vi "Autolocate Fiducials.vi"(6 "FD Index":i32, 8 "error in":errorcluster, 9 "Past Fiducials":dbl[](array[numeric]), 10 "Component":T1, 11 "Gantry In":refnum<k24>) -> (0 "error out":errorcluster, 1 "Wrong Orientation?":bool, 2 "Component Out":T1, 3 "Gantry Out":refnum<k24>)   [LabVIEW 2021, in "Component Tray.lvclass"]
uses:
  Component Tray.lvclass
  C:/Program Files (x86)/Aerotech/A3200/LabVIEW/2010/Bin/Aerotech.A3200.dll
  Program Files (x86)/Aerotech/A3200/LabVIEW/2010/Bin/Aerotech.A3200.dll
  Find Component.ctl
  Controller/Camera/Machine Vision.ctl
  Controller/Motion/A3200/A3200.lvclass
  Controller/Motion/Motion.lvclass
  Controller/Camera/Camera.lvclass
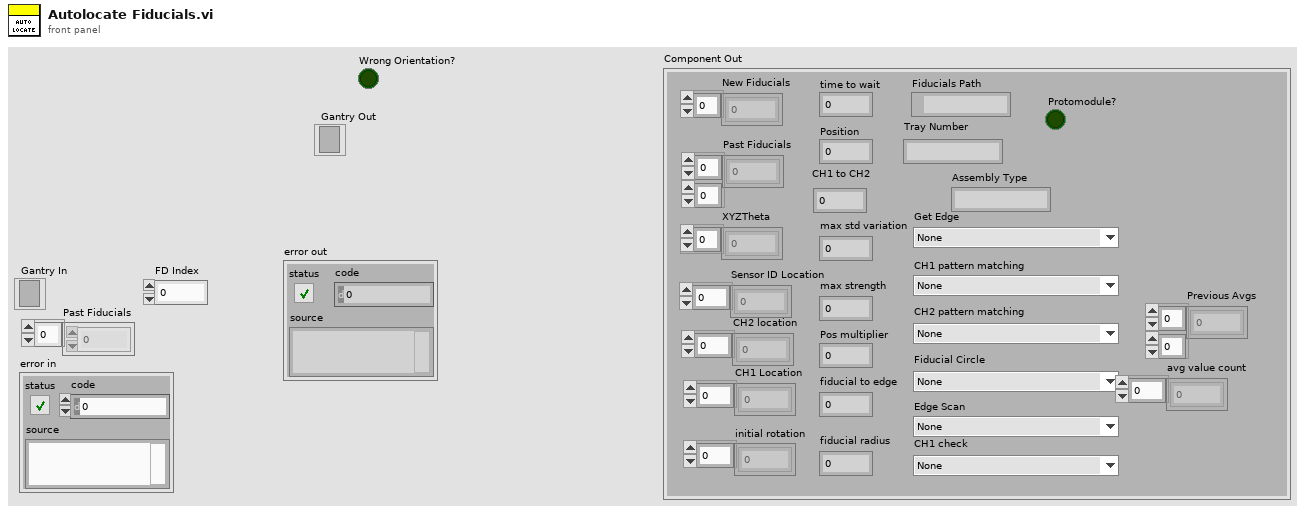
[diagram p1: front panel]
types:
  T1 = typedef "Component Tray.lvclass/Find Component.ctl" = cluster{"New Fiducials":dbl[], "Past Fiducials":dbl[][], "XYZTheta":dbl[], "Fiducials Path":path, "Position":i32, "CH1 Location":dbl[], "Sensor ID Location":dbl[], "initial rotation":dbl[], "CH2 location":dbl[], "max std variation":dbl, "max strength":dbl, "CH2 pattern matching":T2, "Fiducial Circle":T2, "Get Edge":T2, "Pos multiplier":dbl, "time to wait":u32, "fiducial to edge":dbl, "Protomodule?":bool, "Assembly Type":string, "CH1 to CH2":dbl, "Tray Number":string, "fiducial radius":dbl, "4 fiducials?":bool, "CH1 check":T2, "Edge Scan":T2, "CH1 pattern matching":T2, "Sensor Thickness":dbl, "Previous Avgs":dbl[][], "avg value count":dbl[]}
  T2 = typedef "Camera.lvclass/Machine Vision.ctl" = enum16{"None", "Assembly Tray Circle", "Assembly Tray Fiducial", "Partial Hexaboard", "sensor edge init", "HB edge init", "sensor edge pos1", "sensor edge pos2", "HB edge pos1", "HB edge pos2", "Sensor CH1-2", "HB CH1", "HB CH2", "V3 Sensor Circle", "Hexaboard Circle", "sensor CH1 check", "HB CH1 check ", "sensor ID"}
  T3 = enum16{"None", "Assembly Tray Circle", "Assembly Tray Fiducial", "Partial Hexaboard", "sensor edge init", "HB edge init", "sensor edge pos1", "sensor edge pos2", "HB edge pos1", "HB edge pos2", "Sensor CH1-2", "HB CH1", "HB CH2", "V3 Sensor Circle", "Hexaboard Circle", "sensor CH1 check", "HB CH1 check "}
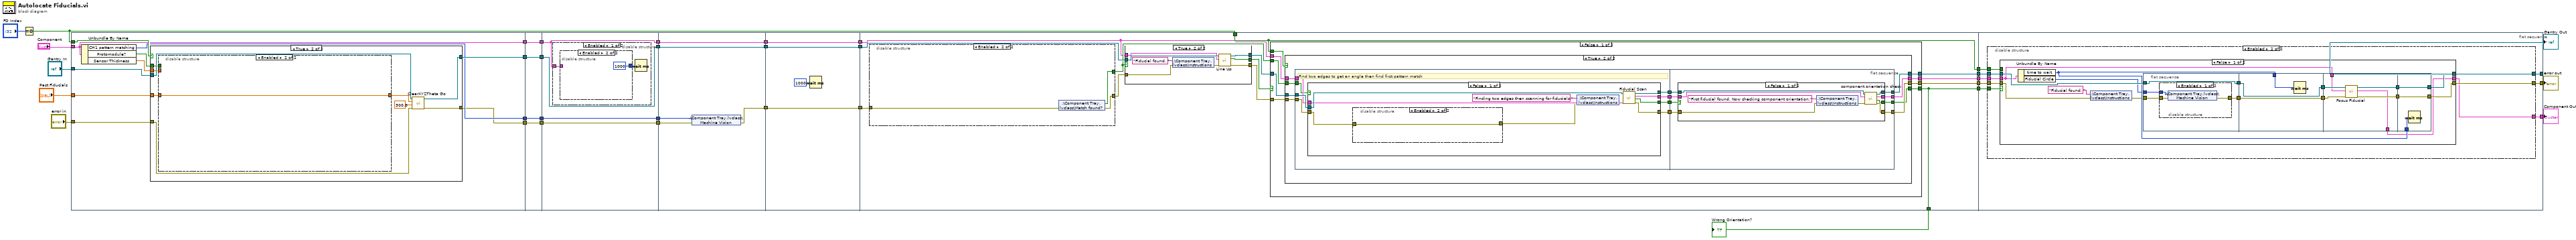
[diagram p0: block diagram]
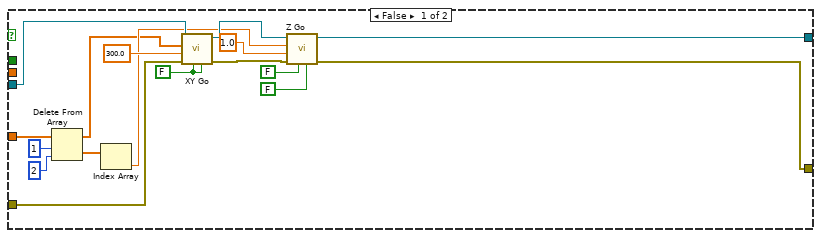
[diagram p2: hidden frame]
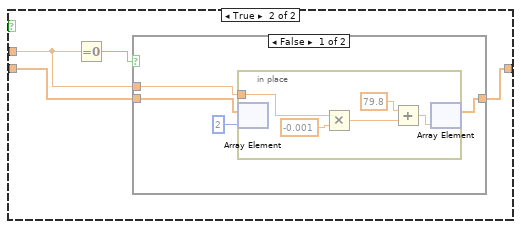
[diagram p4: hidden frame]
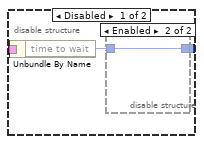
[diagram p6: hidden frame]
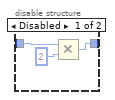
[diagram p7: hidden frame]
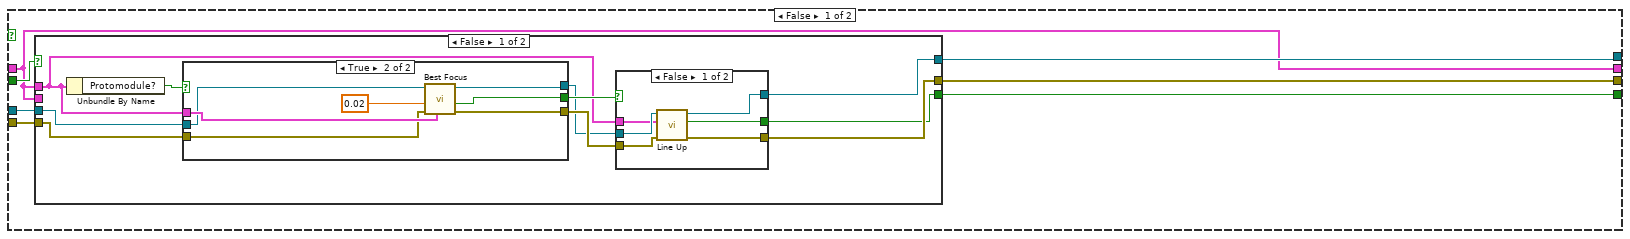
[diagram p9: hidden frame]
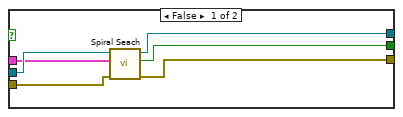
[diagram p10: hidden frame]
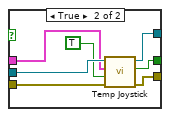
[diagram p11: hidden frame]
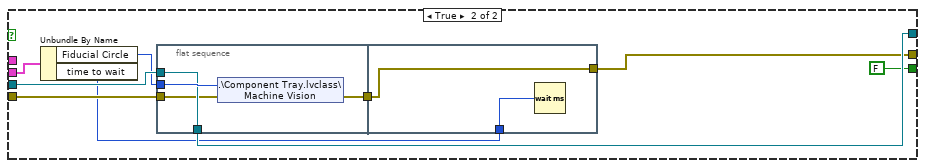
[diagram p12: hidden frame]
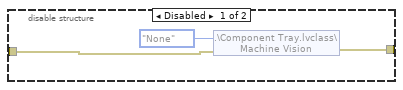
[diagram p13: hidden frame]
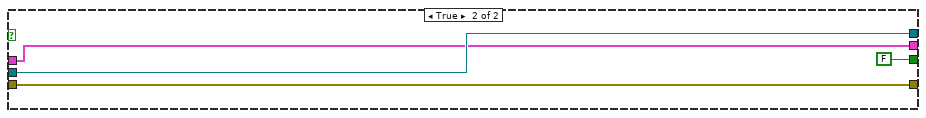
[diagram p14: hidden frame]
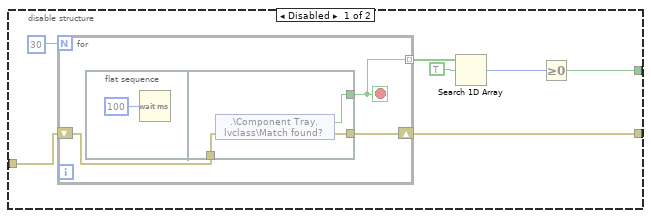
[diagram p17: hidden frame]
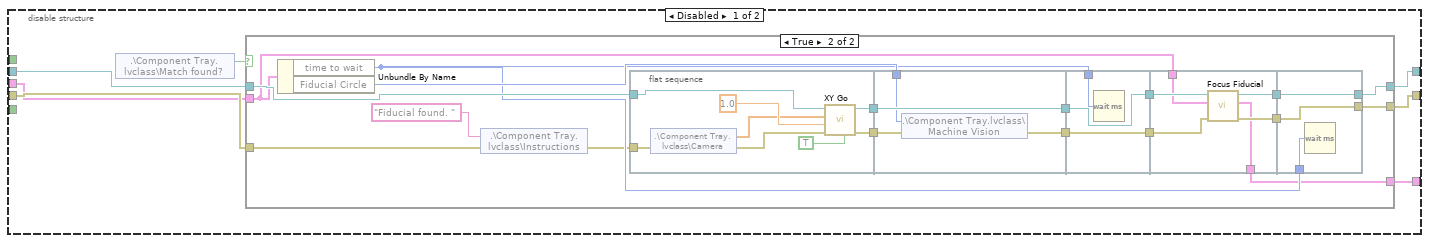
[diagram p19: hidden frame]
diagram:
  n1 = Equal To 0?(x="FD Index") -> (x = 0?=w29:bool)
  n2 = flat-sequence {
    tunnel: w29 -> [w43]
    tunnel: "Gantry In" -> [w42]
    tunnel: "Past Fiducials" -> [w41]
    tunnel: "error in" -> [w36]
    tunnel: [w40] -> w16
    tunnel: "Component" -> [w39]
    tunnel: [w39] -> w18
    tunnel: [w35] -> w10
    tunnel: [w34] -> w7
    tunnel: w18 -> [w93]
    tunnel: [w93] -> w17
    tunnel: w16 -> [w92]
    tunnel: [w92] -> w15
    tunnel: [w91] -> w11
    tunnel: w10 -> [w91]
    tunnel: [w90] -> w8
    tunnel: w7 -> [w90]
    tunnel: w17 -> [w97]
    tunnel: [w97] -> w13
    tunnel: w15 -> [w96]
    tunnel: [w96] -> w14
    tunnel: [w95] -> w12
    tunnel: w11 -> [w95]
    tunnel: [w94] -> w9
    tunnel: w8 -> [w94]
    tunnel: w14 -> [w112]
    tunnel: [w112] -> w6
    tunnel: [w108] -> w4
    tunnel: w13 -> [w111]
    tunnel: [w111] -> w2
    tunnel: w12 -> [w110]
    tunnel: w9 -> [w109]
    tunnel: w6 -> [w116]
    tunnel: [w116] -> w5
    tunnel: w4 -> [w115]
    tunnel: [w115] -> w3
    tunnel: w2 -> [w114]
    tunnel: [w114] -> w1
    tunnel: w29 -> [w125]
    tunnel: [w129] -> w28
    tunnel: [w127] -> w27
    tunnel: [w128] -> w25
    tunnel: [w126] -> w24
    tunnel: [w126] -> w23
    tunnel: [w125] -> w22
    tunnel: w5 -> [w121]
    tunnel: w3 -> [w124]
    tunnel: w1 -> [w118]
    tunnel: [w295] -> w19
    tunnel: [w294] -> w21
    tunnel: w28 -> [w293]
    tunnel: w27 -> [w291]
    tunnel: [w290] -> w20
    tunnel: w25 -> [w292]
    tunnel: w23 -> [w289]
    tunnel: w22 -> [w288]
    frame #0 {
      n3 = Unbundle By Name(w39) -> ("CH1 pattern matching"=w35:T2, "Protomodule?"=w38:bool, "Sensor Thickness"=w37:dbl)
      n4 = case shown="True" w43 {
        tunnel: w41 -> [w56 w65]
        tunnel: w42 -> [w60 w69]
        tunnel: [w54 w68] -> w40
        tunnel: w36 -> [w58 w67]
        tunnel: w38 -> [_ w61]
        tunnel: [w53 w66] -> w34
        tunnel: w37 -> [_ w64]
        frame False {
          w59 = FALSE ("Increment?")
          n5 = Delete From Array(array=w56, length=1, index=2) -> (deleted portion=w46:dbl[], array with subset deleted=w44:dbl[])
          n6 = Index Array(array=w46) -> (element=w45:dbl)  [unwired: 1 in]
          n7 = call "XY Go.vi"("Increment?"=w59, "return immediately"=w59, "error in (no error)"=w58, "Speed"=300.0, "XY In"=w44, "Gantry In"=w60) -> ("error out"=w52:errorcluster, "Gantry Out"=w55:refnum<k24>)  [unwired: 3 in, 1 out]
          n8 = call "Z Go.vi"("Increment"=FALSE, "Return Immediately"=FALSE, "error in (no error)"=w52, "Speed In"=1.0, "Position In"=w45, "Gantry In"=w55) -> ("error out"=w53:errorcluster, "Gantry Out"=w54:refnum<k24>)  [unwired: 2 in, 2 out]
        }
        frame True {
          n9 = disable-structure shown="Enabled" {
            disable-tunnel: w65 -> [w73 w89]
            disable-tunnel: w64 -> [w72 _]
            disable-tunnel: [w71 w89] -> w63
            disable-tunnel: w61 -> [w70 _]
            frame Disabled {
              n10 = case shown="False" w70 {
                tunnel: w73 -> [w74 w77]
                tunnel: w72 -> [_ w76]
                tunnel: [w74 w75] -> w71
                frame False {
                }
                frame True {
                  n11 = Equal To 0?(x=w76) -> (x = 0?=w78:bool)
                  n12 = case shown="False" w78 {
                    tunnel: w77 -> [w82 w88]
                    tunnel: w76 -> [w81 _]
                    tunnel: [w80 w88] -> w75
                    frame False {
                      n13 = in-place {
                        in-place-border: w81 -> [w86]
                        n14 = in-place-array #1(w82, 2) -> ()  [unwired: 1 out]
                        n15 = Multiply(x=w86, y=-0.001) -> (x*y=w84:dbl)
                        n16 = Add(x=79.8, y=w84) -> (x+y=w83:dbl)
                        n17 = in-place-array #1(w83) -> (w80:dbl[])  [unwired: 1 out]
                      }
                    }
                    frame True {
                    }
                  }
                }
              }
            }
            frame Enabled {
            }
          }
          n18 = call "ClearXYZTheta Go.vi"("error in (no error)"=w67, "Speed"=300.0, "XYZTheta In"=w63, "Gantry In"=w69) -> ("error out"=w66:errorcluster, "Gantry Out"=w68:refnum<k24>)  [unwired: 5 in, 1 out]
        }
      }
    }
    frame #1 {
    }
    frame #2 {
      n19 = disable-structure shown="Enabled" {
        disable-tunnel: w97 -> [w99 _]
        frame Enabled {
          n20 = disable-structure shown="Enabled" {
            disable-tunnel: w99 -> [w102 _]
            disable-tunnel: [w100 u32 1000 ("time to wait")] -> w98
            frame Disabled {
              n21 = Unbundle By Name(w102) -> ("time to wait"=w101:u32)
              n22 = disable-structure shown="Enabled" {
                disable-tunnel: w101 -> [w105 w106]
                disable-tunnel: [w103 w106] -> w100
                frame Disabled {
                  n23 = Multiply(x=w105, y=u32 2) -> (x*y=w103:u32)
                }
                frame Enabled {
                }
              }
            }
            frame Enabled {
            }
          }
          n24 = Wait (ms)(milliseconds to wait=w98) -> ()  [unwired: 1 out]
        }
        frame Disabled {
        }
      }
    }
    frame #3 {
      n25 = shared-variable ".\\Component Tray.lvclass\\Machine Vision"(w110, error in=w109) -> (error out=w108:errorcluster)
    }
    frame #4 {
      n26 = Wait (ms)(milliseconds to wait=u32 1000) -> ()  [unwired: 1 out]
    }
    frame #5 {
      n27 = disable-structure shown="Enabled" {
        disable-tunnel: w124 -> [w266 w275]
        disable-tunnel: [w264 w276] -> w123
        disable-tunnel: [w260 w274] -> w119
        frame Disabled {
          n28 = for {
            N: 30 -> [_]
            tunnel: [w268] -> w263 mode=indexing
            shift-right: [w267] -> w264
            shift-left: w266 -> [w269]
            stop <- w268 stop-if-true
            n29 = flat-sequence {
              tunnel: w269 -> [w273]
              tunnel: [w272] -> w268
              tunnel: [w271] -> w267
              frame #0 {
                n30 = Wait (ms)(milliseconds to wait=u32 100) -> ()  [unwired: 1 out]
              }
              frame #1 {
                n31 = shared-variable ".\\Component Tray.lvclass\\Match found?"(error in=w273) -> (w272:bool, error out=w271:errorcluster)
              }
            }
          }
          n32 = Search 1D Array(1D array=w263, element=TRUE) -> (index of element=w261:i32)  [unwired: 1 in]
          n33 = Greater Or Equal To 0?(x=w261) -> (x >= 0?=w260:bool)
        }
        frame Enabled {
          n34 = shared-variable ".\\Component Tray.lvclass\\Match found?"(error in=w275) -> (w274:bool, error out=w276:errorcluster)
        }
      }
      n35 = case shown="True" w119 {
        selector: w119 -> [w277 _]
        tunnel: w123 -> [w279 w286]
        tunnel: [w279 w282] -> w122
        tunnel: w121 -> [w278 w285]
        tunnel: [w278 w284] -> w120
        tunnel: w118 -> [_ w281]
        tunnel: [w277 w280] -> w117
        frame False {
        }
        frame True {
          n36 = shared-variable ".\\Component Tray.lvclass\\Instructions"("Fiducial found. " ("Instructions"), error in=w286) -> (error out=w283:errorcluster)
          n37 = call "Line Up.vi"("error IO"=w283, "Component"=w281, "Gantry In"=w285) -> ("error out"=w282:errorcluster, "Error?"=w280:bool, "Gantry Out"=w284:refnum<k24>)  [unwired: 6 in]
        }
      }
      n38 = case shown="False" w117 {
        selector: w117 -> [_ w257]
        tunnel: [w138 w259] -> w129
        tunnel: [w137 w258] -> w128
        tunnel: [w136 w256] -> w127
        tunnel: [w135 w257] -> w126
        tunnel: w125 -> [w134 _]
        tunnel: w122 -> [w133 w258]
        tunnel: w120 -> [w132 w259]
        tunnel: w119 -> [w131 _]
        tunnel: w118 -> [w130 w256]
        frame False {
          n39 = case shown="True" w134 {
            tunnel: w132 -> [w145 w208]
            tunnel: [w144 w207] -> w138
            tunnel: [w143 w206] -> w137
            tunnel: w130 -> [w139 w205]
            tunnel: [w139 w204] -> w136
            tunnel: [w140 w200] -> w135
            tunnel: w131 -> [w141 w198]
            tunnel: w133 -> [w142 w197]
            frame False {
              n40 = case shown="False" w141 {
                tunnel: w142 -> [w152 w190]
                tunnel: w145 -> [w151 w189]
                tunnel: w139 -> [_ w187]
                tunnel: [w155 w188] -> w144
                tunnel: [w154 w185] -> w143
                tunnel: [w146 FALSE ("Wrong Orientation?")] -> w140
                tunnel: w139 -> [w147 _]
                frame False {
                  n41 = Unbundle By Name(w147) -> ("Protomodule?"=w153:bool)
                  n42 = case shown="True" w153 {
                    tunnel: w147 -> [w156 w168]
                    tunnel: w152 -> [w157 w167]
                    tunnel: w151 -> [w161 w166]
                    tunnel: [w158 w165] -> w150
                    tunnel: [w159 w164] -> w149
                    tunnel: [w160 w163] -> w148
                    frame False {
                      n43 = call "Spiral Seach.vi"("error in (no error)"=w157, "Component"=w156, "Gantry In"=w161) -> ("error out"=w158:errorcluster, "Error?"=w159:bool, "Gantry Out"=w160:refnum<k24>)  [unwired: 6 in]
                    }
                    frame True {
                      n44 = call "Best Focus.vi"("Component"=w168, "error in (no error)"=w167, "Inc by"=0.02 ("Start"), "Gantry In"=w166) -> ("error out"=w165:errorcluster, "Error?"=w164:bool, "Gantry Out"=w163:refnum<k24>)  [unwired: 4 in, 1 out]
                    }
                  }
                  n45 = case shown="False" w149 {
                    tunnel: w148 -> [w174 w181]
                    tunnel: [w173 w180] -> w155
                    tunnel: [w172 w176] -> w154
                    tunnel: w150 -> [w171 w177]
                    tunnel: w147 -> [w170 w179]
                    tunnel: [w169 w175] -> w146
                    frame False {
                      n46 = call "Line Up.vi"("error IO"=w171, "Component"=w170, "Gantry In"=w174) -> ("error out"=w172:errorcluster, "Error?"=w169:bool, "Gantry Out"=w173:refnum<k24>)  [unwired: 6 in]
                    }
                    frame True {
                      n47 = call "Temp Joystick.vi"("error in (no error)"=w177, "Fiducial?"=TRUE, "Component"=w179, "Gantry In"=w181) -> ("error out"=w176:errorcluster, "Error?"=w175:bool, "Gantry Out"=w180:refnum<k24>)  [unwired: 5 in]
                    }
                  }
                }
                frame True {
                  n48 = Unbundle By Name(w187) -> ("Fiducial Circle"=w186:T2, "time to wait"=w183:u32)
                  n49 = flat-sequence {
                    tunnel: w186 -> [w194]
                    tunnel: [w193] -> w184
                    tunnel: w190 -> [w191]
                    tunnel: [w192] -> w188
                    tunnel: w189 -> [w192]
                    tunnel: [w196] -> w185
                    tunnel: w184 -> [w196]
                    tunnel: w183 -> [w195]
                    frame #0 {
                      n50 = shared-variable ".\\Component Tray.lvclass\\Machine Vision"(w194, error in=w191) -> (error out=w193:errorcluster)
                    }
                    frame #1 {
                      n51 = Wait (ms)(milliseconds to wait=w195) -> ()  [unwired: 1 out]
                    }
                  }
                }
              }
            }
            frame True {
              n52 = flat-sequence {
                tunnel: w208 -> [w216]
                tunnel: w205 -> [w213]
                tunnel: [w215] -> w203
                tunnel: [w214] -> w202
                tunnel: [w212] -> w201
                tunnel: [w211] -> w199
                tunnel: w198 -> [w210]
                tunnel: w197 -> [w209]
                tunnel: [w239] -> w204
                tunnel: [w241] -> w206
                tunnel: [w242] -> w207
                tunnel: [w240] -> w200
                tunnel: w201 -> [w236]
                tunnel: w202 -> [w237]
                tunnel: w203 -> [w238]
                tunnel: w199 -> [w235]
                frame #0 {
                  # "Find two edges to get an angle then find first pattern match"
                  n53 = case shown="False" w210 {
                    tunnel: w216 -> [w226 w234]
                    tunnel: [w225 w234] -> w215
                    tunnel: w209 -> [w219 w233]
                    tunnel: [w224 w233] -> w214
                    tunnel: w213 -> [w223 w232]
                    tunnel: [w222 w232] -> w212
                    tunnel: [w221 FALSE] -> w211
                    frame False {
                      n54 = disable-structure shown="Enabled" {
                        disable-tunnel: w219 -> [w228 w230]
                        disable-tunnel: [w227 w230] -> w218
                        frame Disabled {
                          n55 = shared-variable ".\\Component Tray.lvclass\\Machine Vision"(T3."None" ("Machine Vision"), error in=w228) -> (error out=w227:errorcluster)
                        }
                        frame Enabled {
                        }
                      }
                      n56 = shared-variable ".\\Component Tray.lvclass\\Instructions"("Finding two edges then scanning for fiducials." ("Instructions"), error in=w218) -> (error out=w217:errorcluster)
                      n57 = call "Fiducial Scan.vi"("error in"=w217, "input cluster"=w223, "Gantry In"=w226) -> ("error out"=w224:errorcluster, "Not Found?"=w221:bool, "output cluster"=w222:T1, "Gantry Out"=w225:refnum<k24>)  [unwired: 5 in]
                    }
                    frame True {
                    }
                  }
                }
                frame #1 {
                  n58 = case shown="False" w235 {
                    selector: w235 -> [_ w252]
                    tunnel: [w251 w255] -> w242
                    tunnel: [w250 w253] -> w241
                    tunnel: [w249 w252] -> w240
                    tunnel: [w248 w254] -> w239
                    tunnel: w238 -> [w246 w255]
                    tunnel: w237 -> [w244 w253]
                    tunnel: w236 -> [w247 w254]
                    frame False {
                      n59 = shared-variable ".\\Component Tray.lvclass\\Instructions"("First fiducial found. Now checking component orientation." ("Instructions"), error in=w244) -> (error out=w243:errorcluster)
                      n60 = call "component orientation check.vi"("error in"=w243, "input cluster"=w247, "Gantry In"=w246) -> ("error out"=w250:errorcluster, "Wrong Orientation?"=w249:bool, "output cluster"=w248:T1, "Gantry Out"=w251:refnum<k24>)  [unwired: 5 in]
                    }
                    frame True {
                    }
                  }
                }
              }
            }
          }
        }
        frame True {
        }
      }
    }
    frame #6 {
      n61 = disable-structure shown="Enabled" {
        disable-tunnel: [w302 w352] -> w295
        disable-tunnel: [w301 w351] -> w294
        disable-tunnel: w293 -> [w300 w355]
        disable-tunnel: w292 -> [w299 w354]
        disable-tunnel: w291 -> [w298 w353]
        disable-tunnel: [w297 w350] -> w290
        disable-tunnel: w289 -> [_ w349]
        disable-tunnel: w288 -> [_ w348]
        frame Disabled {
          n62 = shared-variable ".\\Component Tray.lvclass\\Match found?"() -> (w296:bool)  [unwired: 1 in, 1 out]
          n63 = case shown="True" w296 {
            tunnel: w300 -> [w305 w323]
            tunnel: [w305 w322] -> w302
            tunnel: w299 -> [w303 w307]
            tunnel: w298 -> [w304 w318]
            tunnel: [w303 w319] -> w301
            tunnel: [w304 w309] -> w297
            frame False {
            }
            frame True {
              n64 = Unbundle By Name(w318) -> ("time to wait"=w310:u32, "Fiducial Circle"=w315:T2)
              n65 = shared-variable ".\\Component Tray.lvclass\\Instructions"("Fiducial found. " ("Instructions"), error in=w307) -> (error out=w306:errorcluster)
              n66 = flat-sequence {
                tunnel: w323 -> [w331]
                tunnel: w306 -> [w325]
                tunnel: [w330] -> w321
                tunnel: [w327] -> w320
                tunnel: w321 -> [w335]
                tunnel: [w335] -> w314
                tunnel: w320 -> [w333]
                tunnel: [w332] -> w312
                tunnel: w315 -> [w334]
                tunnel: w314 -> [w338]
                tunnel: [w338] -> w313
                tunnel: w312 -> [w337]
                tunnel: [w337] -> w311
                tunnel: w310 -> [w336]
                tunnel: w313 -> [w342]
                tunnel: w311 -> [w341]
                tunnel: w318 -> [w340]
                tunnel: [w344] -> w317
                tunnel: [w343] -> w316
                tunnel: [w339] -> w309
                tunnel: [w346] -> w319
                tunnel: [w347] -> w322
                tunnel: w317 -> [w347]
                tunnel: w316 -> [w346]
                tunnel: w310 -> [w345]
                frame #0 {
                  n67 = shared-variable ".\\Component Tray.lvclass\\Camera"(error in=w325) -> (w326:dbl[], error out=w324:errorcluster)
                  n68 = call "XY Go.vi"("Increment?"=TRUE, "error in (no error)"=w324, "Speed"=1.0, "XY In"=w326, "Gantry In"=w331) -> ("error out"=w327:errorcluster, "Gantry Out"=w330:refnum<k24>)  [unwired: 4 in, 1 out]
                }
                frame #1 {
                  n69 = shared-variable ".\\Component Tray.lvclass\\Machine Vision"(w334, error in=w333) -> (error out=w332:errorcluster)
                }
                frame #2 {
                  n70 = Wait (ms)(milliseconds to wait=w336) -> ()  [unwired: 1 out]
                }
                frame #3 {
                  n71 = call "Focus Fiducial.vi"("error in"=w341, "Component In"=w340, "Gantry In"=w342) -> ("error out"=w343:errorcluster, "Component Out"=w339:T1, "Gantry Out"=w344:refnum<k24>)  [unwired: 6 in]
                }
                frame #4 {
                  n72 = Wait (ms)(milliseconds to wait=w345) -> ()  [unwired: 1 out]
                }
              }
            }
          }
        }
        frame Enabled {
          n73 = case shown="False" w349 {
            tunnel: w355 -> [w371 w394]
            tunnel: [w370 w394] -> w352
            tunnel: w354 -> [w357 w392]
            tunnel: w353 -> [w368 w393]
            tunnel: [w369 w392] -> w351
            tunnel: [w360 w393] -> w350
            tunnel: w348 -> [_ _]
            frame False {
              n74 = Unbundle By Name(w368) -> ("time to wait"=w361:u32, "Fiducial Circle"=w356:T2)
              n75 = shared-variable ".\\Component Tray.lvclass\\Instructions"("Fiducial found. " ("Instructions"), error in=w357) -> (error out=w358:errorcluster)
              n76 = flat-sequence {
                tunnel: [w372] -> w365
                tunnel: [w374] -> w363
                tunnel: w356 -> [w375]
                tunnel: w358 -> [w373]
                tunnel: w371 -> [w372]
                tunnel: w365 -> [w382]
                tunnel: [w382] -> w364
                tunnel: w363 -> [w381]
                tunnel: [w381] -> w362
                tunnel: w361 -> [w380]
                tunnel: w364 -> [w386]
                tunnel: w362 -> [w385]
                tunnel: w368 -> [w384]
                tunnel: [w388] -> w367
                tunnel: [w387] -> w366
                tunnel: [w383] -> w360
                tunnel: [w390] -> w369
                tunnel: [w391] -> w370
                tunnel: w367 -> [w391]
                tunnel: w366 -> [w390]
                tunnel: w361 -> [w389]
                frame #0 {
                  n77 = disable-structure shown="Enabled" {
                    disable-tunnel: w375 -> [w378 _]
                    disable-tunnel: w373 -> [w377 w379]
                    disable-tunnel: [w376 w379] -> w374
                    frame Enabled {
                      n78 = shared-variable ".\\Component Tray.lvclass\\Machine Vision"(w378, error in=w377) -> (error out=w376:errorcluster)
                    }
                    frame Disabled {
                    }
                  }
                }
                frame #1 {
                  n79 = Wait (ms)(milliseconds to wait=w380) -> ()  [unwired: 1 out]
                }
                frame #2 {
                  n80 = call "Focus Fiducial.vi"("error in"=w385, "Component In"=w384, "Gantry In"=w386) -> ("error out"=w387:errorcluster, "Component Out"=w383:T1, "Gantry Out"=w388:refnum<k24>)  [unwired: 6 in]
                }
                frame #3 {
                  n81 = Wait (ms)(milliseconds to wait=w389) -> ()  [unwired: 1 out]
                }
              }
            }
            frame True {
            }
          }
        }
      }
    }
  }
  "Gantry Out" <- w19
  "error out" <- w21
  "Component Out" <- w20
  "Wrong Orientation?" <- w24
